vi "write-point.vi"(7 "dvr":refnum<data-value>, 8 "error in (no error)":errorcluster, 10 "y_axis":dbl[](array[numeric]), 11 "x_axis":dbl) -> (0 "error out":errorcluster, 3 "index":i32)   [LabVIEW 2015, in "lv-graph-global.lvlib"]
doc: "write can be used to write a single \"set\" of data to the dvr. It's inputs are a single value for the x axis and one or more values for the y axis."
uses:
  lv-graph-global.lvlib
  _controls/data.ctl
  _controls/configuration.ctl
  _controls/store_method.ctl
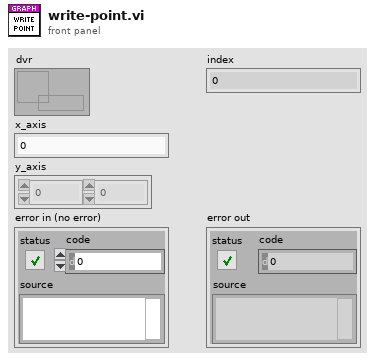
[diagram p1: front panel]
types:
  T1 = typedef "lv-graph-global.lvlib/data.ctl" = cluster{"configuration":T2, "index":i32, "x_axis":dbl[], "y_axis":dbl[][]}
  T2 = typedef "lv-graph-global.lvlib/configuration.ctl" = cluster{"store_method":T3, "rows":i32, "columns":i32}
  T3 = typedef "lv-graph-global.lvlib/store_method.ctl" = enum16{"<store_method>", "fixed", "grow"}
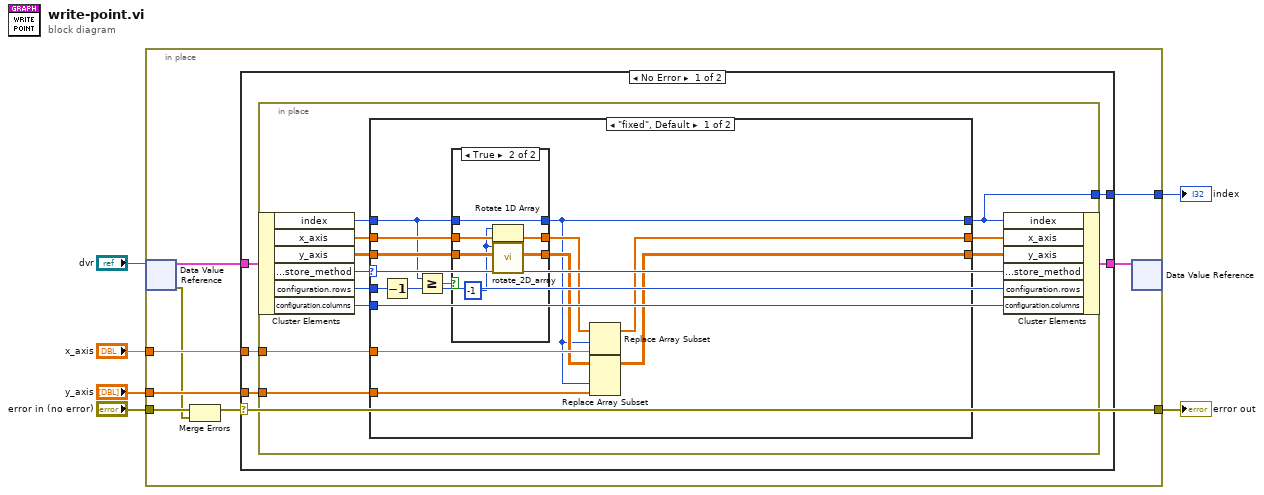
[diagram p0: block diagram]
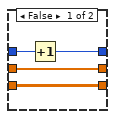
[diagram p2: hidden frame]
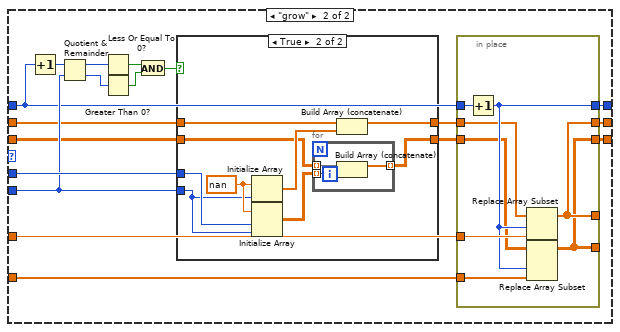
[diagram p3: hidden frame]
diagram:
  n1 = in-place {
    in-place-border: "x_axis" -> [w14]
    in-place-border: "y_axis" -> [w13]
    in-place-border: "error in (no error)" -> [w10]
    in-place-border: [w8] -> w2
    in-place-border: [w7] -> w1
    n2 = in-place-dvr #1("dvr") -> (w11:T1, w9:errorcluster)
    n3 = Merge Errors(w10, w9) -> (w8:errorcluster)
    n4 = case shown="No Error" w8 {
      tunnel: w14 -> [w19 _]
      tunnel: w13 -> [w18 _]
      tunnel: [w17 w94] -> w12
      tunnel: w11 -> [w16 w94]
      tunnel: [w15 _] -> w7
      frame No Error {
        n5 = in-place {
          in-place-border: w19 -> [w30]
          in-place-border: w18 -> [w29]
          in-place-border: [w23] -> w15
          n6 = in-place-cluster #2(w16) -> ("index"=w28:i32, "x_axis"=w27:dbl[], "y_axis"=w26:dbl[][], "configuration.store_method"=w20:T3, "configuration.rows"=w21:i32, "configuration.columns"=w22:i32)
          n7 = case shown="\"fixed\", Default" w20 {
            tunnel: w21 -> [w31 w71]
            tunnel: w22 -> [_ w70]
            tunnel: w30 -> [w43 w69]
            tunnel: w29 -> [w33 w68]
            tunnel: w28 -> [w34 w57]
            tunnel: w27 -> [w36 w61]
            tunnel: w26 -> [w35 w60]
            tunnel: [w38 w55] -> w25
            tunnel: [w32 w54] -> w24
            tunnel: [w37 w56] -> w23
            frame "fixed", Default {
              n8 = Decrement(x=w31) -> (x-1=w42:i32)
              n9 = Greater Or Equal?(x=w34, y=w42) -> (x >= y?=w40:bool)
              n10 = case shown="True" w40 {
                tunnel: w36 -> [w46 w52]
                tunnel: w35 -> [w44 w50]
                tunnel: [w46 w53] -> w39
                tunnel: [w44 w49] -> w41
                tunnel: [w47 w51] -> w37
                tunnel: w34 -> [w45 w51]
                frame False {
                  n11 = Increment(x=w45) -> (x+1=w47:i32)
                }
                frame True {
                  w48 = -1 ("n")
                  n12 = Rotate 1D Array(1:w52, 2:w48) -> (0:w53:dbl[])
                  n13 = call "rotate_2D_array.vi"("array"=w50, "n"=w48) -> ("array_rotated"=w49:dbl[][])  [unwired: 9 in]
                }
              }
              n14 = Replace Array Subset(array=w39, new element=w43, index=w37) -> (w38:dbl[])
              n15 = Replace Array Subset(array=w41, new element=w33, index (col)=w37) -> (w32:dbl[][])  [unwired: 1 in]
            }
            frame "grow" {
              n16 = Increment(x=w57) -> (x+1=w67:i32)
              n17 = Quotient & Remainder(x=w67, y=w70) -> (x-y*floor(x/y)=w65:i32, floor(x/y)=w66:i32)
              n18 = Less Or Equal To 0?(x=w65) -> (x <= 0?=w63:bool)
              n19 = Greater Than 0?(x=w66) -> (x > 0?=w64:bool)
              n20 = And(x=w63, y=w64) -> (x .and. y?=w62:bool)
              n21 = case shown="True" w62 {
                tunnel: w70 -> [_ w79]
                tunnel: w71 -> [_ w80]
                tunnel: w61 -> [w73 w77]
                tunnel: w60 -> [w72 w76]
                tunnel: [w73 w75] -> w59
                tunnel: [w72 w74] -> w58
                frame False {
                }
                frame True {
                  w82 = nan ("element")
                  n22 = Initialize Array(w82, w79) -> (w81:dbl[])
                  n23 = Initialize Array(w82, w80, w79) -> (w78:dbl[][])
                  n24 = for {
                    tunnel: w76 -> [w85] mode=indexing
                    tunnel: w78 -> [w84] mode=indexing
                    tunnel: [w83] -> w74 mode=indexing
                    n25 = Build Array (concatenate)(w85, w84) -> (w83:dbl[])
                  }
                  n26 = Build Array (concatenate)(w77, w81) -> (w75:dbl[])
                }
              }
              n27 = in-place {
                in-place-border: w69 -> [w93]
                in-place-border: w68 -> [w92]
                in-place-border: [w91] -> w56
                in-place-border: [w87] -> _
                in-place-border: [w86] -> _
                in-place-border: w59 -> [w90]
                in-place-border: w58 -> [w89]
                in-place-border: w57 -> [w88]
                in-place-border: [w87] -> w55
                in-place-border: [w86] -> w54
                n28 = Increment(x=w88) -> (x+1=w91:i32)
                n29 = Replace Array Subset(array=w90, new element=w93, index=w91) -> (w87:dbl[])
                n30 = Replace Array Subset(array=w89, new element=w92, index (col)=w91) -> (w86:dbl[][])  [unwired: 1 in]
              }
            }
          }
          n31 = in-place-cluster #2("index"=w23, "x_axis"=w25, "y_axis"=w24, "configuration.store_method"=w20, "configuration.rows"=w21, "configuration.columns"=w22) -> (w17:T1)
        }
      }
      frame Error {
      }
    }
    n32 = in-place-dvr #1(w12) -> ()  [unwired: 2 out]
  }
  "error out" <- w2
  "index" <- w1
